vi "Tosca-Get TTL Queues.vi"(0 "Devices in":refnum<class "TTLControlledDevice.lvclass">[](array[class]), 11 "error in (no error)":errorcluster) -> (4 "Devices out":refnum<class "TTLControlledDevice.lvclass">[](array[class]), 8 "Queues":refnum<queue>[](array[refnum]), 15 "error out":errorcluster)   [LabVIEW 2020]
uses:
  Device Classes/Base Class/TTLControlledDevice.lvclass
  D:/Experiment VIs/Koop/KObject Class/KObject.lvclass
  Control Classes/Base Class/TTLController.lvclass
  Device Classes/Base Class/TTLControlledDevice.lvclass/TTLControlledDevice.ctl
  Control Classes/TTLWaterController/TTLWaterController.lvclass
  D:/Experiment VIs/Tosca/LV Source/TTL VIs/Control Classes/Base Class/TTLController.lvclass
  Device Classes/Base Class/Read Name.vi
  epl-vi-lib/Koop/KObject Class/KObject.lvclass
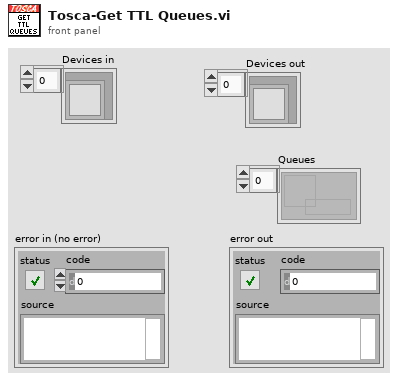
[diagram p1: front panel]
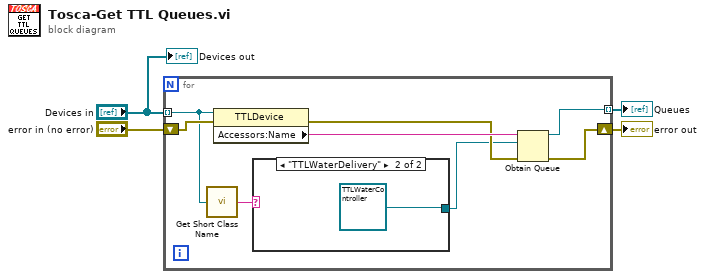
[diagram p0: block diagram]
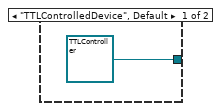
[diagram p2: hidden frame]
diagram:
  n1 = for {
    tunnel: "Devices in" -> [w10] mode=indexing
    shift-right: [w8] -> w1
    shift-left: "error in (no error)" -> [w11]
    tunnel: [w7] -> w2 mode=indexing
    n2 = call "Get Short Class Name.vi"("KObject in"=w10) -> ("Class"=w6:string)  [unwired: 4 in]
    n3 = property class="TTLDevice"(reference=w10, error in=w11) -> (error out=w9:errorcluster, "Accessors:Name"=w12:string)  [unwired: 1 out]
    n4 = case shown="\"TTLWaterDelivery\"" w6 {
      tunnel: [refnum<class "TTLController.lvclass"> refnum ("TTLControl") refnum<class "TTLWaterController.lvclass"> refnum ("TTLWater")] -> w5
      frame "TTLControlledDevice", Default {
      }
      frame "TTLWaterDelivery" {
      }
    }
    n5 = Obtain Queue(name (unnamed)=w12, element data type=w5, error in (no error)=w9) -> (queue out=w7:refnum<queue>, error out=w8:errorcluster)  [unwired: 2 in, 1 out]
  }
  "Queues" <- w2
  "error out" <- w1
  "Devices out" <- "Devices in"
